vi "ni579x Configure LO Filter.vi"(0 "Register Bus":T1, 1 "scope":string(combo)="rx", 5 "frequency [Hz]":dbl format="%#_6p", 11 "Error In":errorcluster) -> (4 "Register Bus (out)":T1, 6 "coerced frequency [Hz]":dbl format="%#_6p", 15 "Error Out":errorcluster)   [LabVIEW 2015, in "ni579x Config v2 Host.lvlib"]
uses:
  <instrlib>/ni579x/Config/v2/Host/ni579x Config v2 Host.lvlib
  <instrlib>/_niInstr/Register Bus/v0/Host/Public/Register Bus Session.ctl
  <instrlib>/_niInstr/Register Bus/v0/Host/Private/Session Data.ctl
  <instrlib>/_niInstr/Register Bus/v0/Host/niInstr Register Bus v0 Host.lvlib
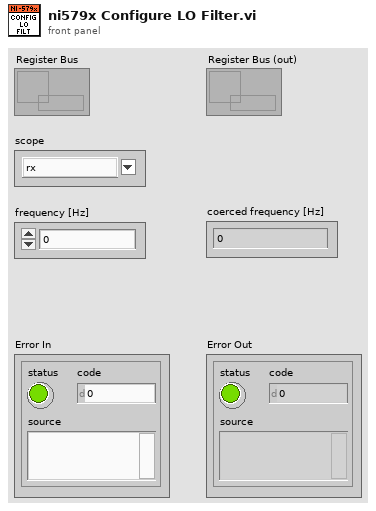
[diagram p1: front panel]
types:
  T1 = typedef "niInstr Register Bus v0 Host.lvlib/Register Bus Session.ctl" = refnum<queue>
  T2 = typedef "ni579x Config v2 Shared.lvlib/ni579x User Command.ctl" = cluster{"User Data 0":u8, "User Data 1":u8, "User Command ID":T3}
  T3 = typedef "ni579x Config v2 Shared.lvlib/ni579x User Command ID.ctl" = u8
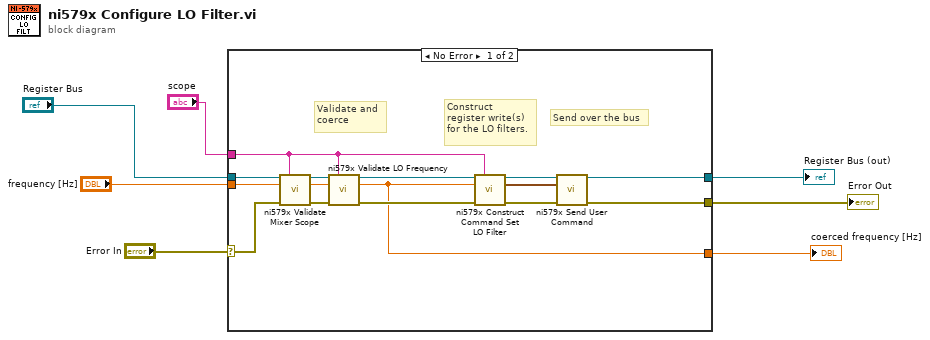
[diagram p0: block diagram]
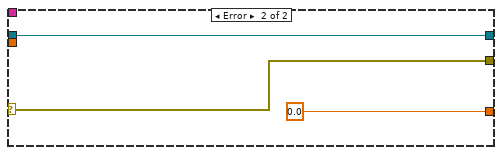
[diagram p2: hidden frame]
diagram:
  n1 = case shown="No Error" "Error In" {
    selector: "Error In" -> [w10 w24]
    tunnel: [w19 w24] -> w6
    tunnel: "Register Bus" -> [w12 w23]
    tunnel: "frequency [Hz]" -> [w21 _]
    tunnel: [w20 w23] -> w3
    tunnel: [w13 0.0 ("coerced attenuation [dB]")] -> w2
    tunnel: "scope" -> [w8 _]
    frame No Error {
      # "Construct\nregister write(s)\nfor the LO filters."
      # "Send over the bus"
      # "Validate and \ncoerce"
      n2 = call <instrlib>:"ni579x Validate Mixer Scope.vi"("Register Bus"=w12, "scope"=w8, "Error In"=w10) -> ("Register Bus (out)"=w11:T1, "Error Out"=w9:errorcluster)  [unwired: 11 in]
      n3 = call <instrlib>:"ni579x Validate LO Frequency.vi"("Register Bus"=w11, "scope"=w8, "frequency [Hz]"=w21, "Error In"=w9) -> ("Register Bus (out)"=w15:T1, "coerced frequency [Hz]"=w13:dbl, "Error Out"=w14:errorcluster)  [unwired: 9 in]
      n4 = call <instrlib>:"ni579x Construct Command Set LO Filter.vi"("Register Bus"=w15, "scope"=w8, "frequency [Hz]"=w13, "Error In"=w14) -> ("Register Bus (out)"=w18:T1, "User Command"=w17:T2, "Error Out"=w16:errorcluster)  [unwired: 9 in]
      n5 = call <instrlib>:"ni579x Send User Command.vi"("Register Bus"=w18, "User Command"=w17, "Error In"=w16) -> ("Register Bus (out)"=w20:T1, "Error Out"=w19:errorcluster)  [unwired: 8 in, 3 out]
    }
    frame Error {
    }
  }
  "Register Bus (out)" <- w3
  "Error Out" <- w6
  "coerced frequency [Hz]" <- w2
